vi "CH375_Get.vi"() -> (2 "当前状态":bool, 3 "当前角度":dbl)   [LabVIEW 2020]
uses:
  Global_CH375.vi
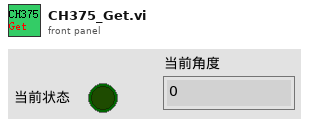
[diagram p1: front panel]
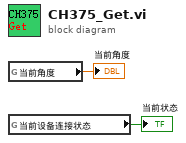
[diagram p0: block diagram]
diagram:
  n1 = global read "Global_CH375.vi" "当前角度"() -> (→"当前角度":dbl)
  n2 = global read "Global_CH375.vi" "当前设备连接状态"() -> (→"当前状态":bool)
